vi "Dontula_Exercise2Task3.vi"() -> ()   [LabVIEW 2014, in "Dontula_3_Ex2Task1_12-6-16.lvrbt"]
uses:
  Dontula_3_Ex2Task1_12-6-16.lvrbt
panel:
  out "Average Value":dbl
  out "Waveform Graph":dynamicdata(graph)
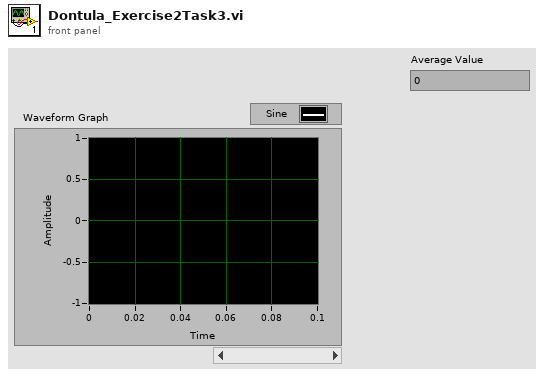
[diagram p1: front panel]
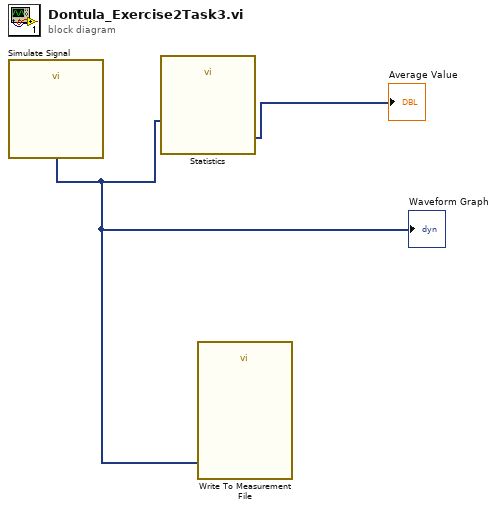
[diagram p0: block diagram]
diagram:
  n1 = call "Simulate Signal"() -> ("Sine"=w2:dynamicdata)  [unwired: 14 in, 1 out]
  "Waveform Graph" <- w2
  n2 = call "Statistics"("Signals"=w2) -> ("Arithmetic Mean"=→"Average Value":dynamicdata)  [unwired: 25 in, 1 out]
  n3 = call "Write To Measurement File"("Signals"=w2) -> ()  [unwired: 16 in, 3 out]
